vi "User & System Details.vi"() -> (2 "Boolean":bool, 5 "User Name 2":string caption="שם משתמש", 7 "מספר סידורי 2":string caption="מספר סידורי")   [LabVIEW 2015]
uses:
  <vilib>/Utility/file.llb/Read From Spreadsheet File (string).vi
  <vilib>/Utility/file.llb/Write To Spreadsheet File (string).vi
panel:
  in  "Cancel Button":bool
  in  "Next Button":bool
  in  "User Name":string caption="שם משתמש"
  in  "מספר סידורי":string
  out "Msg":string
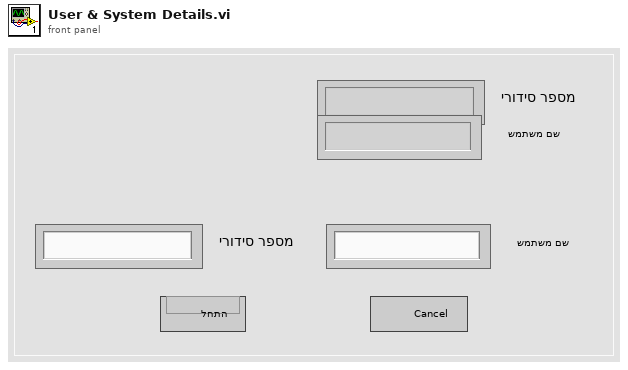
[diagram p1: front panel]
types:
  T1 = enum32{"Invalid", "Standard", "Closed", "Hidden", "Minimized", "Maximized"}
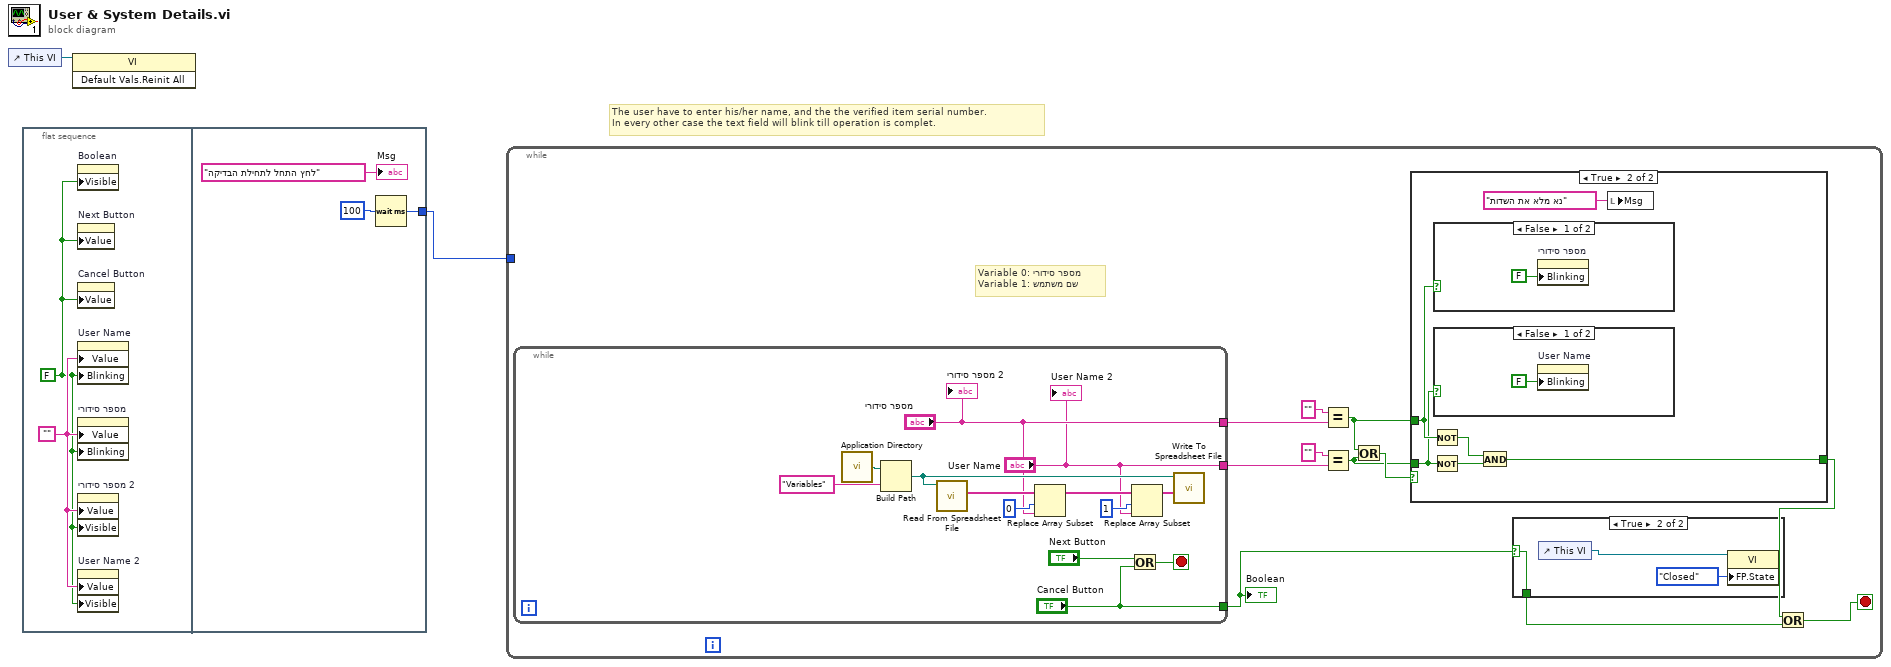
[diagram p0: block diagram]
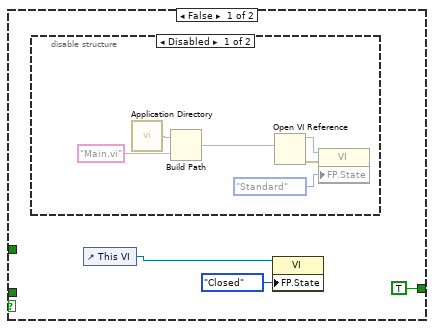
[diagram p3: hidden frame]
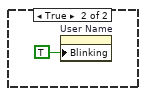
[diagram p5: hidden frame]
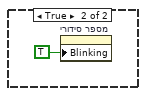
[diagram p6: hidden frame]
diagram:
  # "The user have to enter his/her name, and the the verified item serial number.\nIn every other case the text field will blink till operation is complet."
  n1 = control-ref of="This VI"() -> (w1:refnum<vi>)
  n2 = flat-sequence {
    tunnel: [w6] -> w2
    frame #0 {
      w4 = ""
      w3 = FALSE
      n3 = property on="Boolean" class="Bool (strict)"("Visible"=w3) -> ()  [unwired: 2 in, 2 out]
      n4 = property on="Next Button" class="Bool (strict)"("Value"=w3) -> ()  [unwired: 2 in, 2 out]
      n5 = property on="Cancel Button" class="Bool (strict)"("Value"=w3) -> ()  [unwired: 2 in, 2 out]
      n6 = property on="User Name" class="Str"("Value"=w4, "Blinking"=w3) -> ()  [unwired: 2 in, 2 out]
      n7 = property on="מספר סידורי" class="Str"("Value"=w4, "Blinking"=w3) -> ()  [unwired: 2 in, 2 out]
      n8 = property on="מספר סידורי 2" class="Str"("Value"=w4, "Visible"=w3) -> ()  [unwired: 2 in, 2 out]
      n9 = property on="User Name 2" class="Str"("Value"=w4, "Visible"=w3) -> ()  [unwired: 2 in, 2 out]
    }
    frame #1 {
      n10 = Wait (ms)(milliseconds to wait=u32 100) -> (millisecond timer value=w6:u32)
      "Msg" <- "לחץ התחל לתחילת הבדיקה" ("mainMsg")
    }
  }
  n11 = invoke class="VI" method="Default Vals.Reinit All"(reference=w1) -> ()  [unwired: 2 in, 3 out]
  n12 = while {
    tunnel: w2 -> [_]
    stop <- w10 stop-if-true
    # "Variable 0: מספר סידורי\nVariable 1: שם משתמש"
    n13 = while {
      tunnel: ["מספר סידורי"] -> w13
      tunnel: ["User Name"] -> w12
      tunnel: ["Cancel Button"] -> w9
      stop <- w43 stop-if-true
      n14 = call <vilib>:"Application Directory.vi"() -> ("Application Directory"=w53:path)
      n15 = Build Path(base path=w53, name or relative path="Variables") -> (appended path=w51:path)
      n16 = call-poly <vilib>:"Read From Spreadsheet File.vi"("file path (dialog if empty)"=w51) -> ("first row"=w52:string[])  [unwired: 6 in, 4 out]
      n17 = Replace Array Subset(array=w52, new element="מספר סידורי", index=0) -> (w47:string[])
      n18 = Or(x="Next Button", y="Cancel Button") -> (x .or. y?=w43:bool)
      n19 = Replace Array Subset(array=w47, new element="User Name", index=1) -> (w48:string[])
      n20 = call-poly <vilib>:"Write To Spreadsheet File.vi"("1D data"=w48, "file path (dialog if empty)"=w51) -> ()  [unwired: 6 in, 1 out]
      "מספר סידורי 2" <- "מספר סידורי"
      "User Name 2" <- "User Name"
    }
    "Boolean" <- w9
    n21 = Equal?(x="", y=w13) -> (x = y?=w16:bool)
    n22 = Equal?(x="", y=w12) -> (x = y?=w17:bool)
    n23 = Or(x=w16, y=w17) -> (x .or. y?=w18:bool)
    n24 = case shown="True" w18 {
      tunnel: w16 -> [_ w37]
      tunnel: w17 -> [_ w36]
      tunnel: [TRUE w32] -> w11
      frame False {
        n25 = disable-structure shown="Disabled" {
          frame Disabled {
            n26 = call <vilib>:"Application Directory.vi"() -> ("Application Directory"=w30:path)
            n27 = Build Path(base path=w30, name or relative path="Main.vi") -> (appended path=w31:path)
            n28 = Open VI Reference(vi path=w31) -> (vi reference=w28:refnum<vi>, error out=w27:errorcluster)  [unwired: 5 in]
            n29 = property class="VI"(reference=w28, error in=w27, "FP.State"=T1."Standard" ("Front Panel Window:State")) -> ()  [unwired: 2 out]
          }
          frame Enabled {
          }
        }
        n30 = control-ref of="This VI"() -> (w24:refnum<vi>)
        n31 = property class="VI"(reference=w24, "FP.State"=T1."Closed" ("Front Panel Window:State")) -> ()  [unwired: 1 in, 2 out]
      }
      frame True {
        n32 = Not(x=w37) -> (.not. x?=w35:bool)
        n33 = Not(x=w36) -> (.not. x?=w34:bool)
        n34 = case shown="False" w37 {
          frame False {
            n35 = property on="מספר סידורי" class="Str"("Blinking"=FALSE) -> ()  [unwired: 2 in, 2 out]
          }
          frame True {
            n36 = property on="מספר סידורי" class="Str"("Blinking"=TRUE) -> ()  [unwired: 2 in, 2 out]
          }
        }
        n37 = case shown="False" w36 {
          frame False {
            n38 = property on="User Name" class="Str"("Blinking"=FALSE) -> ()  [unwired: 2 in, 2 out]
          }
          frame True {
            n39 = property on="User Name" class="Str"("Blinking"=TRUE) -> ()  [unwired: 2 in, 2 out]
          }
        }
        n40 = And(x=w35, y=w34) -> (x .and. y?=w32:bool)
        n41 = local write "Msg"("נא מלא את השדות" ("Msg")) -> ()
      }
    }
    n42 = case shown="True" w9 {
      selector: w9 -> [w19 w22]
      tunnel: [w19 w22] -> w8
      frame False {
      }
      frame True {
        n43 = control-ref of="This VI"() -> (w20:refnum<vi>)
        n44 = property class="VI"(reference=w20, "FP.State"=T1."Closed" ("Front Panel Window:State")) -> ()  [unwired: 1 in, 2 out]
      }
    }
    n45 = Or(x=w11, y=w8) -> (x .or. y?=w10:bool)
  }
